vi "NI-DAQmx_Create.vi"(0 "reference in":refnum<class "NI-DAQmx.lvclass">, 1 "AI Task":refnum<k21>, 2 "DO Task":refnum<k21>, 3 "AO Task":refnum<k21>, 5 "error in (no error)":errorcluster) -> (13 "ProcessViRef":refnum<vi>, 14 "reference out":refnum<class "NI-DAQmx.lvclass">, 19 "error out":errorcluster)   [LabVIEW 2020, in "NI-DAQmx.lvclass"]
uses:
  NI-DAQmx.lvclass
  controls/IO Signal List.ctl
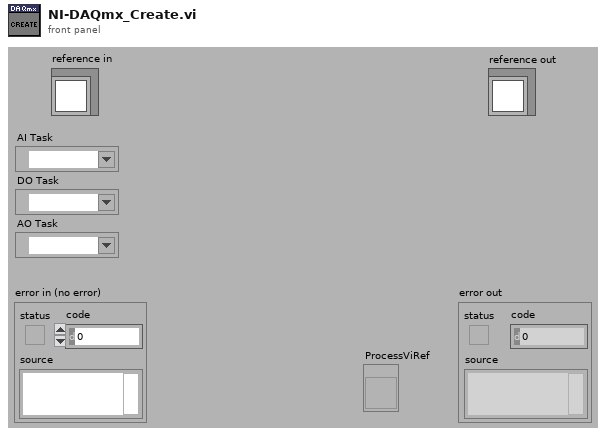
[diagram p1: front panel]
types:
  T1 = typedef "IO Signal List.ctl" = enum16{"Timestamp", "PSU_FB_U_VDC", "PSU_FB_I_AMP", "PSU_FB_W_WATT", "PSU_CMD_U_VDC", "PSU_CMD_I_AMP", "PSU_CMD_OUTPUT", "LCR_PRIMARY", "LCR_SECONDARY", "UV_R_Ohm", "UW_R_Ohm", "VW_R_Ohm", "UV_L_H", "UW_L_H", "VW_L_H", "U_U_VDC", "V_U_VDC", "W_U_VDC", "U_I_AMP", "V_I_AMP", "W_I_AMP", "PWM_CMD_DC_%", "PWM_CMD_VDC", "PWM_CMD_Hz", "PWM_FB_DC_%", "PWM_FB_VDC", "PWM_FB_Hz", "DO_RELAY_U_LCR_A", "DO_RELAY_V_LCR_A", "DO_RELAY_V_LCR_B", "DO_RELAY_W_LCR_B", "DIFF_UV_UW_L_H", "DIFF_UV_VW_L_H", "DIFF_UW_VW_L_H", "DIFF_UV_UW_R_Ohm", "DIFF_UV_VW_R_Ohm", "DIFF_UW_VW_R_Ohm", "DIFF_UV_U_VDC", "DIFF_UW_U_VDC", "DIFF_VW_U_VDC"}
  T2 = typedef "NI-DAQmx.lvclass/ObjectAttributes.ctl" = cluster{"AI Task":refnum<k21>, "DO Task":refnum<k21>, "AO Task":refnum<k21>, "Latest Values":dbl[], "Signal List":T1[], "PWM Duty Cycle (%)":dbl, "PWM Amplitude (V)":dbl, "PWM Frequency (Hz)":dbl, "DO States":bool[]}
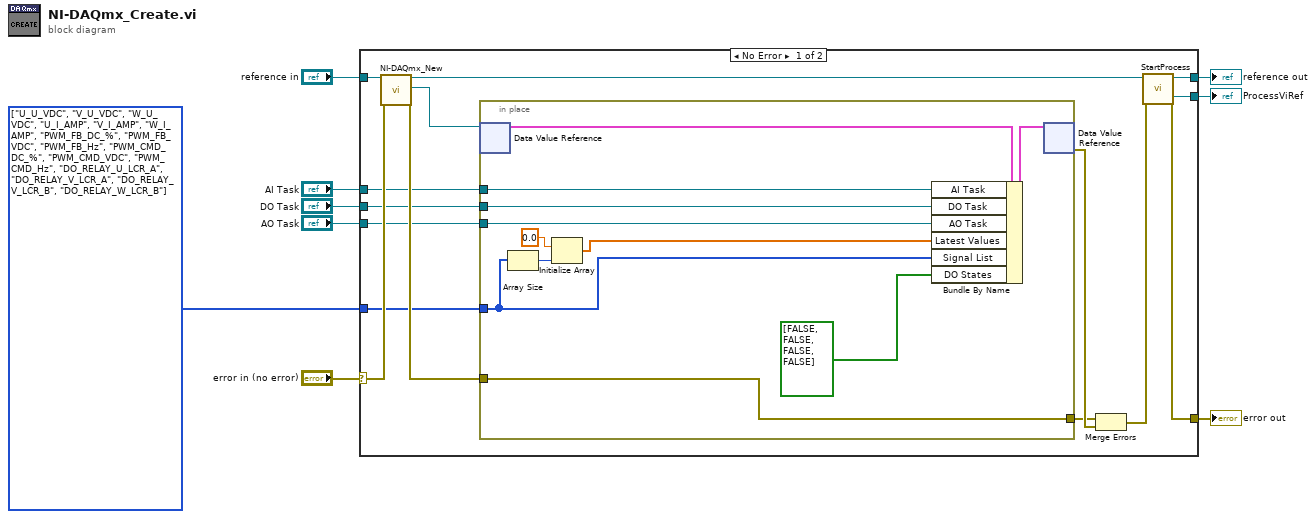
[diagram p0: block diagram]
diagram:
  w1 = T1[] [enum."U_U_VDC", enum."V_U_VDC", enum."W_U_VDC", enum."U_I_AMP", enum."V_I_AMP", enum."W_I_AMP", enum."PWM_FB_DC_%", enum."PWM_FB_VDC", enum."PWM_FB_Hz", enum."PWM_CMD_DC_%", enum."PWM_CMD_VDC", enum."PWM_CMD_Hz", enum."DO_RELAY_U_LCR_A", enum."DO_RELAY_V_LCR_A", enum."DO_RELAY_V_LCR_B", enum."DO_RELAY_W_LCR_B"] items=["Timestamp", "PSU_FB_U_VDC", "PSU_FB_I_AMP", "PSU_FB_W_WATT", "PSU_CMD_U_VDC", "PSU_CMD_I_AMP", "PSU_CMD_OUTPUT", "LCR_PRIMARY", "LCR_SECONDARY", "UV_R_Ohm", "UW_R_Ohm", "VW_R_Ohm", "UV_L_H", "UW_L_H", "VW_L_H", "U_U_VDC", "V_U_VDC", "W_U_VDC", "U_I_AMP", "V_I_AMP", "W_I_AMP", "PWM_CMD_DC_%", "PWM_CMD_VDC", "PWM_CMD_Hz", "PWM_FB_DC_%", "PWM_FB_VDC", "PWM_FB_Hz", "DO_RELAY_U_LCR_A", "DO_RELAY_V_LCR_A", "DO_RELAY_V_LCR_B", "DO_RELAY_W_LCR_B", "DIFF_UV_UW_L_H", "DIFF_UV_VW_L_H", "DIFF_UW_VW_L_H", "DIFF_UV_UW_R_Ohm", "DIFF_UV_VW_R_Ohm", "DIFF_UW_VW_R_Ohm", "DIFF_UV_U_VDC", "DIFF_UW_U_VDC", "DIFF_VW_U_VDC"] ("Data Channels")
  n1 = case shown="No Error" "error in (no error)" {
    selector: "error in (no error)" -> [w23 w37]
    tunnel: [w15 w37] -> w8
    tunnel: "reference in" -> [w24 w36]
    tunnel: [w17 w36] -> w6
    tunnel: [w14 _] -> w5
    tunnel: "AI Task" -> [w13 _]
    tunnel: "DO Task" -> [w12 _]
    tunnel: "AO Task" -> [w11 _]
    tunnel: w1 -> [w10 _]
    frame No Error {
      n2 = call "NI-DAQmx_New.vi"("reference in"=w24, "error in (no error)"=w23) -> ("reference out"=w18:refnum<class "NI-DAQmx.lvclass">, "DVRRefOut"=w21:refnum<data-value>, "error out"=w20:errorcluster)  [unwired: 14 in, 1 out]
      n3 = in-place {
        in-place-border: w20 -> [w26]
        in-place-border: [w26] -> w19
        in-place-border: w13 -> [w27]
        in-place-border: w12 -> [w33]
        in-place-border: w11 -> [w25]
        in-place-border: w10 -> [w32]
        n4 = in-place-dvr #1(w21) -> (w34:T2)  [unwired: 1 out]
        n5 = Array Size(array=w32) -> (size(s)=w31:i32)
        n6 = Initialize Array(0.0 ("element"), w31) -> (w29:dbl[])
        n7 = Bundle By Name(cluster=w34, "AI Task"=w27, "DO Task"=w33, "AO Task"=w25, "Latest Values"=w29, "Signal List"=w32, "DO States"=bool[] [FALSE, FALSE, FALSE, FALSE]) -> (w35:T2)
        n8 = in-place-dvr #1(w35) -> (w22:errorcluster)  [unwired: 1 out]
      }
      n9 = Merge Errors(w19, w22) -> (w16:errorcluster)
      n10 = call "StartProcess.vi"("reference in"=w18, "error in (no error)"=w16) -> ("reference out"=w17:refnum<class "NI-DAQmx.lvclass">, "ProcessViRef"=w14:refnum<vi>, "error out"=w15:errorcluster)  [unwired: 13 in, 2 out]
    }
    frame Error {
      # "VI-TechBaseTemplate_Simple_6x8x6"
    }
  }
  "error out" <- w8
  "reference out" <- w6
  "ProcessViRef" <- w5
